vi "crossandshoot.vi"   [LabVIEW 2015]
uses:
  <vilib>/Rock Robotics/WPI/CAN/TalonSRX/WPI_CANTalonSRX_APIControlMode.ctl
types:
  T1 = typedef "WPI_EncoderDevRef.ctl" = cluster{"DevStatus":errorcluster, "EncoderIndex":T2, "CounterIndex":T3, "DistancePerCount":dbl, "Decoding Type":T4}
  T2 = typedef "FPGA_EncoderIdx.ctl" = enum8{"Enc 0", "Enc 1", "Enc 2", "Enc 3", "Enc 4", "Enc 5", "Enc 6", "Enc 7", "Invalid"}
  T3 = typedef "FPGA_CounterCtrSystemIndex.ctl" = enum8{"Ctr 0", "Ctr 1", "Ctr 2", "Ctr 3", "Ctr 4", "Ctr 5", "Ctr 6", "Ctr 7", "Invalid"}
  T4 = typedef "WPI_EncoderType.ctl" = enum16{"1x", "2x", "4x"}
  T5 = typedef "WPI_MotorControlDeviceRef.ctl" = cluster{"DeviceStatus":errorcluster, "Type":T6, "PWM":cluster{"PWM Channel":T7, "DeadBand":T8}, "CAN":cluster{"Device Number":u8, "Control Mode":T9, "Semaphore":T10, "Max Vout":dbl, "TalonSRX Control Mode":T11}, "Invert":bool}
  T6 = typedef "WPI_MotorControlType.ctl" = enum16{"PWM", "CAN", "CANTalonSRX"}
  T7 = typedef "FPGA_DIOPWMChannel.ctl" = enum8{"PWM 0", "PWM 1", "PWM 2", "PWM 3", "PWM 4", "PWM 5", "PWM 6", "PWM 7", "PWM 8", "PWM 9", "PWM MXP 0", "PWM MXP 1", "PWM MXP 2", "PWM MXP 3", "PWM MXP 4", "PWM MXP 5", "PWM MXP 6", "PWM MXP 7", "PWM MXP 8", "PWM MXP 9", "Invalid"}
  T8 = typedef "WPI_PWMDeadband.ctl" = cluster{"Name":string, "maxPositivePwm":i32, "minPositivePwm":i32, "centerPwm":i32, "maxNegativePwm":i32, "minNegativePwm":i32, "angularRange":u16}
  T9 = typedef "WPI_CANJaguar_ControlMode.ctl" = enum8{"Percent VBus", "Current", "Speed", "Position", "Voltage"}
  T10 = typedef "Semaphore RefNum" = refnum<k1>
  T11 = typedef "WPI_CANTalonSRX_APIControlMode.ctl" = enum8{"Percent VBus", "Speed", "Position", "Slave", "Unchanged / Invalid", "Voltage Compensation", "Current", "Motion Profile"}
  T12 = typedef "WPI_ServoDeviceRef.ctl" = cluster{"DeviceStatus":errorcluster, "PWM Channel":T7, "DeadBand":T8}
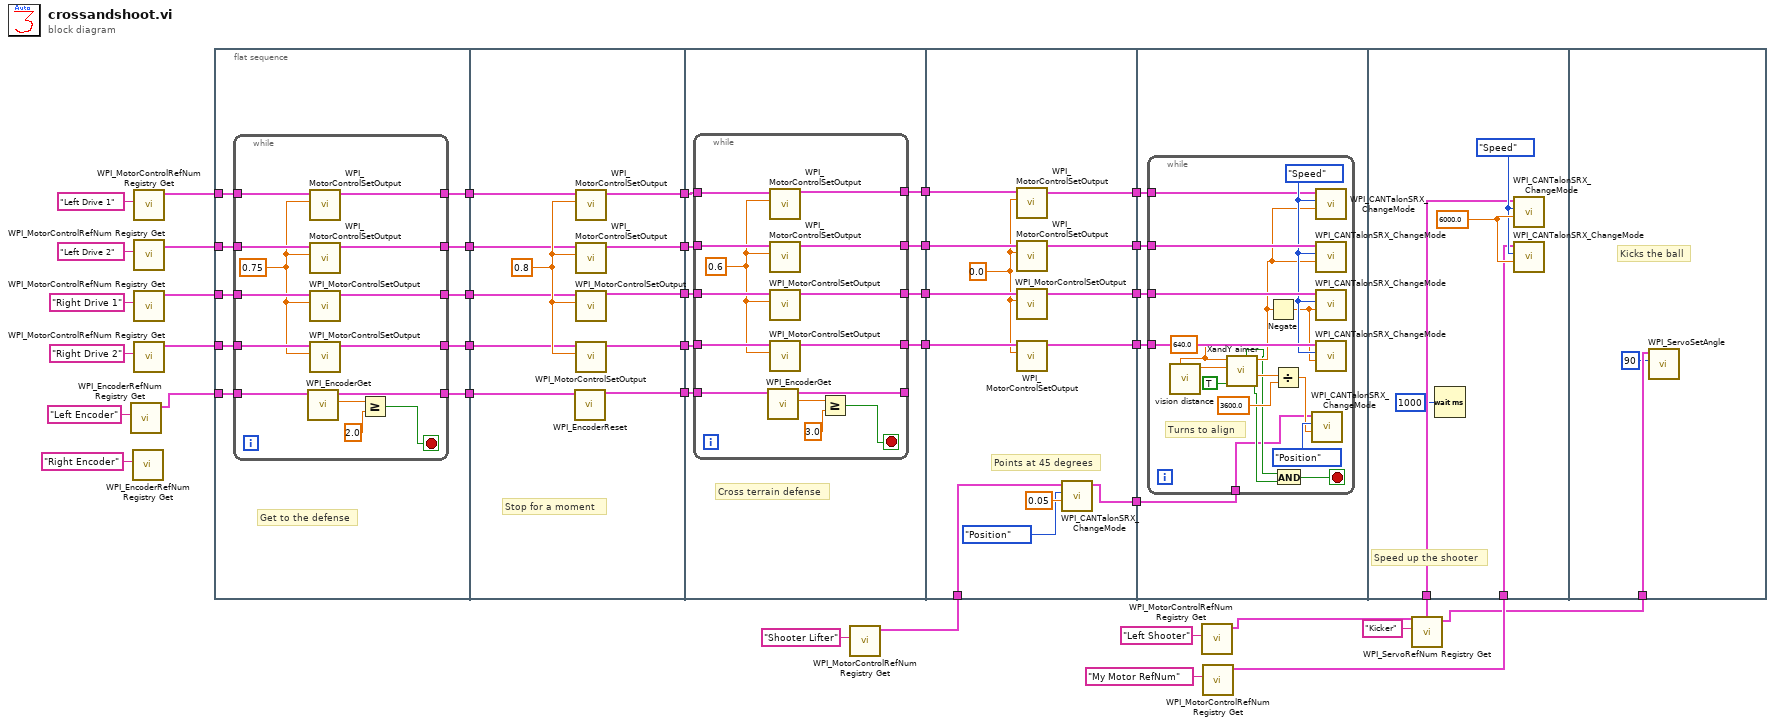
[diagram p0: block diagram]
diagram:
  n1 = call <vilib>:"WPI_EncoderRefNum Registry Get.vi"("refnum name"="Left Encoder") -> ("EncoderDevRef"=w28:T1)  [unwired: 9 in, 1 out]
  n2 = call <vilib>:"WPI_EncoderRefNum Registry Get.vi"("refnum name"="Right Encoder") -> ()  [unwired: 9 in, 2 out]
  n3 = call <vilib>:"WPI_MotorControlRefNum Registry Get.vi"("refnum name"="Left Drive 1") -> ("MotorControlDevRef"=w34:T5)  [unwired: 9 in, 1 out]
  n4 = call <vilib>:"WPI_MotorControlRefNum Registry Get.vi"("refnum name"="Left Drive 2") -> ("MotorControlDevRef"=w33:T5)  [unwired: 9 in, 1 out]
  n5 = call <vilib>:"WPI_MotorControlRefNum Registry Get.vi"("refnum name"="Right Drive 1") -> ("MotorControlDevRef"=w32:T5)  [unwired: 9 in, 1 out]
  n6 = call <vilib>:"WPI_MotorControlRefNum Registry Get.vi"("refnum name"="Right Drive 2") -> ("MotorControlDevRef"=w31:T5)  [unwired: 9 in, 1 out]
  n7 = flat-sequence {
    tunnel: w34 -> [w48]
    tunnel: w33 -> [w47]
    tunnel: w32 -> [w46]
    tunnel: w31 -> [w45]
    tunnel: w28 -> [w44]
    tunnel: [w43] -> w27
    tunnel: [w42] -> w26
    tunnel: [w41] -> w25
    tunnel: [w40] -> w24
    tunnel: [w39] -> w23
    tunnel: w27 -> [w72]
    tunnel: w26 -> [w71]
    tunnel: w25 -> [w70]
    tunnel: w24 -> [w69]
    tunnel: w23 -> [w68]
    tunnel: [w67] -> w22
    tunnel: [w66] -> w21
    tunnel: [w65] -> w20
    tunnel: [w64] -> w19
    tunnel: [w63] -> w18
    tunnel: w22 -> [w82]
    tunnel: w21 -> [w81]
    tunnel: w20 -> [w80]
    tunnel: w19 -> [w79]
    tunnel: w18 -> [w78]
    tunnel: [w77] -> w10
    tunnel: [w76] -> w9
    tunnel: [w75] -> w8
    tunnel: [w74] -> w6
    tunnel: w10 -> [w107]
    tunnel: w9 -> [w103]
    tunnel: w8 -> [w102]
    tunnel: [w109] -> w7
    tunnel: w6 -> [w108]
    tunnel: [w106] -> w5
    tunnel: [w105] -> w4
    tunnel: [w104] -> w3
    tunnel: w2 -> [w98]
    tunnel: [w97] -> w1
    tunnel: w7 -> [w111]
    tunnel: w5 -> [w114]
    tunnel: w4 -> [w112]
    tunnel: w3 -> [w113]
    tunnel: w1 -> [w110]
    tunnel: w16 -> [w135]
    tunnel: w15 -> [w134]
    tunnel: w11 -> [w139]
    frame #0 {
      # "Get to the defense"
      n8 = while {
        tunnel: w48 -> [w62]
        tunnel: w47 -> [w61]
        tunnel: w46 -> [w60]
        tunnel: w45 -> [w59]
        tunnel: w44 -> [w57]
        tunnel: [w53] -> w43
        tunnel: [w52] -> w42
        tunnel: [w51] -> w41
        tunnel: [w50] -> w40
        tunnel: [w49] -> w39
        stop <- w55 stop-if-true
        w58 = 0.75 ("Output")
        n9 = call <vilib>:"WPI_EncoderGet.vi"("EncoderDevRef"=w57) -> ("Distance"=w56:dbl, "EncoderDevRef"=w49:T1)  [unwired: 5 in, 4 out]
        n10 = call <vilib>:"WPI_MotorControlSetOutput.vi"("Output"=w58, "MotorControlDevRef"=w62) -> ("MotorControlDevRef"=w53:T5)  [unwired: 7 in, 2 out]
        n11 = call <vilib>:"WPI_MotorControlSetOutput.vi"("Output"=w58, "MotorControlDevRef"=w61) -> ("MotorControlDevRef"=w52:T5)  [unwired: 7 in, 2 out]
        n12 = call <vilib>:"WPI_MotorControlSetOutput.vi"("Output"=w58, "MotorControlDevRef"=w60) -> ("MotorControlDevRef"=w51:T5)  [unwired: 7 in, 2 out]
        n13 = call <vilib>:"WPI_MotorControlSetOutput.vi"("Output"=w58, "MotorControlDevRef"=w59) -> ("MotorControlDevRef"=w50:T5)  [unwired: 7 in, 2 out]
        n14 = Greater Or Equal?(x=w56, y=2.0) -> (x >= y?=w55:bool)
      }
    }
    frame #1 {
      w73 = 0.8 ("Output")
      # "Stop for a moment"
      n15 = call <vilib>:"WPI_EncoderReset.vi"("EncoderDevRef"=w68) -> ("EncoderDevRef"=w63:T1)  [unwired: 9 in, 1 out]
      n16 = call <vilib>:"WPI_MotorControlSetOutput.vi"("Output"=w73, "MotorControlDevRef"=w72) -> ("MotorControlDevRef"=w67:T5)  [unwired: 7 in, 2 out]
      n17 = call <vilib>:"WPI_MotorControlSetOutput.vi"("Output"=w73, "MotorControlDevRef"=w71) -> ("MotorControlDevRef"=w66:T5)  [unwired: 7 in, 2 out]
      n18 = call <vilib>:"WPI_MotorControlSetOutput.vi"("Output"=w73, "MotorControlDevRef"=w70) -> ("MotorControlDevRef"=w65:T5)  [unwired: 7 in, 2 out]
      n19 = call <vilib>:"WPI_MotorControlSetOutput.vi"("Output"=w73, "MotorControlDevRef"=w69) -> ("MotorControlDevRef"=w64:T5)  [unwired: 7 in, 2 out]
    }
    frame #2 {
      # "Cross terrain defense"
      n20 = while {
        tunnel: w82 -> [w96]
        tunnel: w81 -> [w95]
        tunnel: w80 -> [w94]
        tunnel: w79 -> [w93]
        tunnel: w78 -> [w91]
        tunnel: [w87] -> w77
        tunnel: [w86] -> w76
        tunnel: [w85] -> w75
        tunnel: [w84] -> _
        tunnel: [w83] -> w74
        stop <- w89 stop-if-true
        w92 = 0.6 ("Output")
        n21 = call <vilib>:"WPI_EncoderGet.vi"("EncoderDevRef"=w91) -> ("Distance"=w90:dbl, "EncoderDevRef"=w84:T1)  [unwired: 5 in, 4 out]
        n22 = call <vilib>:"WPI_MotorControlSetOutput.vi"("Output"=w92, "MotorControlDevRef"=w96) -> ("MotorControlDevRef"=w83:T5)  [unwired: 7 in, 2 out]
        n23 = call <vilib>:"WPI_MotorControlSetOutput.vi"("Output"=w92, "MotorControlDevRef"=w95) -> ("MotorControlDevRef"=w87:T5)  [unwired: 7 in, 2 out]
        n24 = call <vilib>:"WPI_MotorControlSetOutput.vi"("Output"=w92, "MotorControlDevRef"=w94) -> ("MotorControlDevRef"=w86:T5)  [unwired: 7 in, 2 out]
        n25 = call <vilib>:"WPI_MotorControlSetOutput.vi"("Output"=w92, "MotorControlDevRef"=w93) -> ("MotorControlDevRef"=w85:T5)  [unwired: 7 in, 2 out]
        n26 = Greater Or Equal?(x=w90, y=3.0) -> (x >= y?=w89:bool)
      }
    }
    frame #3 {
      w101 = 0.0
      # "Points at 45 degrees"
      n27 = call <vilib>:"WPI_MotorControlSetOutput.vi"("Output"=w101, "MotorControlDevRef"=w108) -> ("MotorControlDevRef"=w109:T5)  [unwired: 7 in, 2 out]
      n28 = call <vilib>:"WPI_MotorControlSetOutput.vi"("Output"=w101, "MotorControlDevRef"=w107) -> ("MotorControlDevRef"=w106:T5)  [unwired: 7 in, 2 out]
      n29 = call <vilib>:"WPI_MotorControlSetOutput.vi"("Output"=w101, "MotorControlDevRef"=w103) -> ("MotorControlDevRef"=w104:T5)  [unwired: 7 in, 2 out]
      n30 = call <vilib>:"WPI_MotorControlSetOutput.vi"("Output"=w101, "MotorControlDevRef"=w102) -> ("MotorControlDevRef"=w105:T5)  [unwired: 7 in, 2 out]
      n31 = call <vilib>:"WPI_CANTalonSRX_ChangeMode.vi"("Output"=0.05, "Control Mode"=WPI_CANTalonSRX_APIControlMode."Position", "CAN Talon SRX Ref"=w98) -> ("CAN Talon SRX Ref"=w97:T5)  [unwired: 7 in, 1 out]
    }
    frame #4 {
      n32 = while {
        tunnel: w114 -> [w132]
        tunnel: w113 -> [w131]
        tunnel: w112 -> [w130]
        tunnel: w110 -> [w116]
        tunnel: w111 -> [w115]
        stop <- w119 stop-if-true
        w126 = 640.0
        w129 = WPI_CANTalonSRX_APIControlMode."Speed" ("Control Mode")
        # "Turns to align"
        n33 = call "vision distance.vi"("Image width"=w126) -> ("Distance"=w127:dbl)  [unwired: 10 in]
        n34 = call "XandY aimer.vi"("Aiming?"=TRUE, "Distance"=w127, "Image width"=w126) -> ("Good enough?"=w117:bool, "Y-setpoint"=w122:dbl, "X setpoint"=w124:dbl, "Aiming?"=w118:bool)  [unwired: 5 in]
        n35 = Negate(x=w124) -> (-x=w128:dbl)
        n36 = Divide(x=w122, y=3600.0) -> (x/y=w120:dbl)
        n37 = And(x=w118, y=w117) -> (x .and. y?=w119:bool)
        n38 = call <vilib>:"WPI_CANTalonSRX_ChangeMode.vi"("Output"=w120, "Control Mode"=WPI_CANTalonSRX_APIControlMode."Position", "CAN Talon SRX Ref"=w116) -> ()  [unwired: 7 in, 2 out]
        n39 = call <vilib>:"WPI_CANTalonSRX_ChangeMode.vi"("Output"=w124, "Control Mode"=w129, "CAN Talon SRX Ref"=w115) -> ()  [unwired: 7 in, 2 out]
        n40 = call <vilib>:"WPI_CANTalonSRX_ChangeMode.vi"("Output"=w124, "Control Mode"=w129, "CAN Talon SRX Ref"=w132) -> ()  [unwired: 7 in, 2 out]
        n41 = call <vilib>:"WPI_CANTalonSRX_ChangeMode.vi"("Output"=w128, "Control Mode"=w129, "CAN Talon SRX Ref"=w131) -> ()  [unwired: 7 in, 2 out]
        n42 = call <vilib>:"WPI_CANTalonSRX_ChangeMode.vi"("Output"=w128, "Control Mode"=w129, "CAN Talon SRX Ref"=w130) -> ()  [unwired: 7 in, 2 out]
      }
    }
    frame #5 {
      w136 = WPI_CANTalonSRX_APIControlMode."Speed" ("Control Mode")
      w137 = 6000.0 ("Output")
      # "Speed up the shooter"
      n43 = Wait (ms)(milliseconds to wait=u32 1000) -> ()  [unwired: 1 out]
      n44 = call <vilib>:"WPI_CANTalonSRX_ChangeMode.vi"("Output"=w137, "Control Mode"=w136, "CAN Talon SRX Ref"=w135) -> ()  [unwired: 7 in, 2 out]
      n45 = call <vilib>:"WPI_CANTalonSRX_ChangeMode.vi"("Output"=w137, "Control Mode"=w136, "CAN Talon SRX Ref"=w134) -> ()  [unwired: 7 in, 2 out]
    }
    frame #6 {
      # "Kicks the ball"
      n46 = call <vilib>:"WPI_ServoSetAngle.vi"("Angle"=90, "ServoDeviceRef"=w139) -> ()  [unwired: 8 in, 2 out]
    }
  }
  n47 = call <vilib>:"WPI_MotorControlRefNum Registry Get.vi"("refnum name"="Shooter Lifter") -> ("MotorControlDevRef"=w2:T5)  [unwired: 9 in, 1 out]
  n48 = call <vilib>:"WPI_MotorControlRefNum Registry Get.vi"("refnum name"="Left Shooter") -> ("MotorControlDevRef"=w16:T5)  [unwired: 9 in, 1 out]
  n49 = call <vilib>:"WPI_MotorControlRefNum Registry Get.vi"("refnum name"="My Motor RefNum") -> ("MotorControlDevRef"=w15:T5)  [unwired: 9 in, 1 out]
  n50 = call <vilib>:"WPI_ServoRefNum Registry Get.vi"("refnum name"="Kicker") -> ("ServoDeviceRef"=w11:T12)  [unwired: 9 in, 1 out]
